vi "Get Path.vi"(8 "error in (no error)":errorcluster, 11 "URI in":refnum<class "URI.lvclass">) -> (0 "error out":errorcluster, 2 "path":string, 3 "URI out":refnum<class "URI.lvclass">)   [LabVIEW 2013, in "openURI.lvlib" / "URI.lvclass"]
uses:
  URI.lvclass
  URI.lvclass/URI.ctl
  components/path/URI-Component.Path.lvclass
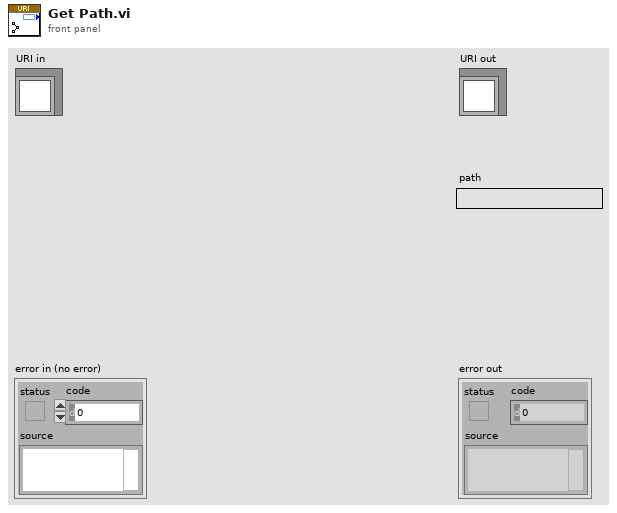
[diagram p1: front panel]
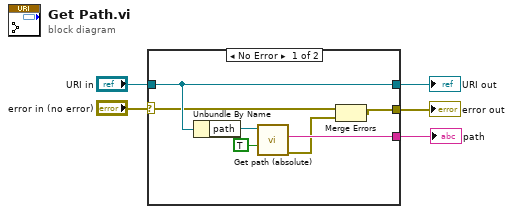
[diagram p0: block diagram]
diagram:
  n1 = case shown="No Error" "error in (no error)" {
    selector: "error in (no error)" -> [w9 w14]
    tunnel: [w7 w14] -> w4
    tunnel: [w10 w13] -> w2
    tunnel: "URI in" -> [w10 w13]
    tunnel: [w11 _] -> w1
    frame No Error {
      n2 = Unbundle By Name(w10) -> ("path"=w12:refnum<class "URI-Component.Path.lvclass">)
      n3 = call "Get path (absolute).vi"("Encoded? (F)"=TRUE, "URI-Component.Path in"=w12) -> ("error out"=w8:errorcluster, "path-component"=w11:string)  [unwired: 7 in, 1 out]
      n4 = Merge Errors(w9, w8) -> (w7:errorcluster)
    }
    frame Error {
    }
  }
  "error out" <- w4
  "URI out" <- w2
  "path" <- w1
